vi "示波器new.vi"() -> ()   [LabVIEW 2018]
uses:
  Tektronix DPO MSO 2000 4000 Series/Tektronix DPO MSO 2000 4000 Series.lvlib
panel:
  out "Waveform Graph":waveform(dbl)(graph)
  in  "Trigger Level (0.0 V)":dbl
  in  "Timebase (0.0005 s)":dbl=0.0005 format="%#_13g"
  in  "电压 范围":dbl=10.0 format="%#_13g"
  in  "偏置 (0.0 V)":dbl
  in  "VISA Resource Name":refnum<visa-resource-name>="TCPIP::192.168.129.100::INSTR"
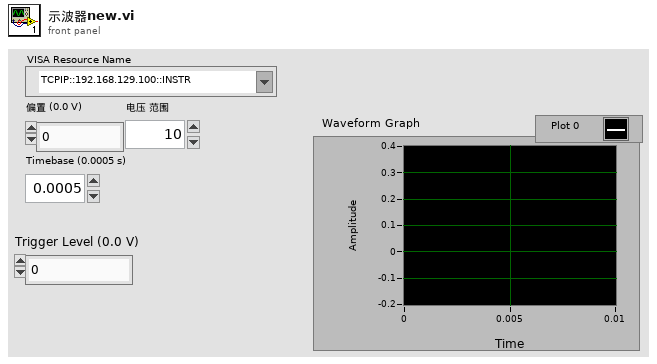
[diagram p1: front panel]
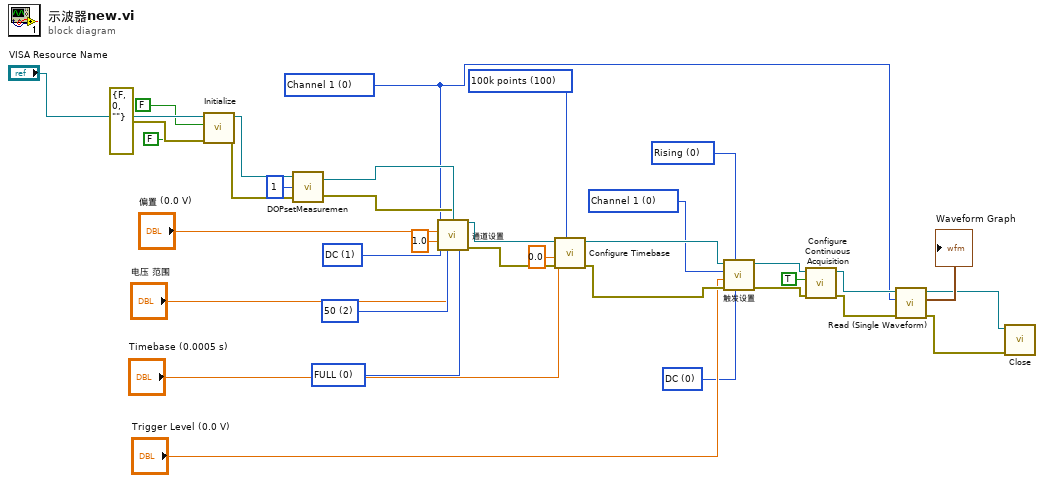
[diagram p0: block diagram]
diagram:
  w10 = u16 0 items=["DC", "HF Reject", "LF Reject", "Noise Reject", "AC"] ("Trigger Coupling (0 : DC)")
  w11 = u16 0 items=["Rising", "Falling", "Either"] ("Trigger Slope (0: Rising)")
  w13 = u16 0 items=["Channel 1", "Channel 2", "Channel 3", "Channel 4", "AC Line", "Aux", "Digital Channel 0", "Digital Channel 1", "Digital Channel 2", "Digital Channel 3", "Digital Channel 4", "Digital Channel 5", "Digital Channel 6", "Digital Channel 7", "Digital Channel 8", "Digital Channel 9", "Digital Channel 10", "Digital Channel 11", "Digital Channel 12", "Digital Channel 13", "Digital Channel 14", "Digital Channel 15", "RF"] ("Trigger Source (0: Channel 1)")
  w16 = u32 100 items=["1000 points"=1, "10k points"=10, "100k points"=100, "1M points"=1000, "5M points"=5000, "10M points"=10000] ("Record Length (10: 10k points)")
  w21 = u16 0 items=["FULL", "250 MHz", "150 MHz", "20 MHz"] ("带宽 (0: FULL)")
  w23 = u16 2 items=["1M", "75", "50"] ("输入阻抗 (0: 1M ohm)")
  w24 = u16 1 items=["AC", "DC", "Ground"] ("耦合(1: DC)")
  w4 = u16 0 items=["Channel 1", "Channel 2", "Channel 3", "Channel 4", "Math", "Reference 1", "Reference 2", "Reference 3", "Reference 4", "Bus 1", "Bus 2"] ("Channel (0: Channel 1)")
  n1 = call "Initialize.vi"("error in (no error)"=errorcluster {"status"=FALSE, "code"=0, "source"=""}, "Reset (True)"=FALSE, "ID Query (True)"=FALSE, "VISA resource name"="VISA Resource Name") -> ("error out"=w30:errorcluster, "VISA resource name out"=w31:refnum<visa-resource-name>)  [unwired: 6 in]
  n2 = call "DOPsetMeasuremen.vi"("error in (no error)"=w30, "CH"=u8 1, "VISA resource name"=w31) -> ("error out"=w27:errorcluster, "VISA resource name out"=w28:refnum<visa-resource-name>)
  n3 = call "通道设置.vi"("Channel (0: Channel 1)"=w4, "范围 (10.0 V)"="电压 范围", "VISA resource name"=w28, "带宽 (0: FULL)"=w21, "偏置 (0.0 V)"="偏置 (0.0 V)", "衰减 (1)"=1.0, "耦合(1: DC)"=w24, "输入阻抗 (0: 1M ohm)"=w23, "error in (no error)"=w27) -> ("VISA resource name out"=w20:refnum<visa-resource-name>, "error out"=w19:errorcluster)  [unwired: 5 in]
  n4 = call "Configure Timebase.vi"("Record Length (10: 10k points)"=w16, "error in (no error)"=w19, "Position (10 %)"=0.0, "Timebase (0.0005 s)"="Timebase (0.0005 s)", "VISA resource name"=w20) -> ("error out"=w14:errorcluster, "VISA resource name out"=w15:refnum<visa-resource-name>)  [unwired: 5 in]
  n5 = call "触发设置.vi"("Trigger Coupling (0 : DC)"=w10, "Trigger Slope (0: Rising)"=w11, "error in (no error)"=w14, "Trigger Level (0.0 V)"="Trigger Level (0.0 V)", "Trigger Source (0: Channel 1)"=w13, "VISA resource name"=w15) -> ("error out"=w8:errorcluster, "VISA resource name out"=w9:refnum<visa-resource-name>)  [unwired: 4 in]
  n6 = call "Configure Continuous Acquisition.vi"("error in (no error)"=w8, "Enable Continuous Acquisition Mode (T: Enable)"=TRUE, "VISA resource name"=w9) -> ("error out"=w5:errorcluster, "VISA resource name out"=w6:refnum<visa-resource-name>)  [unwired: 7 in]
  n7 = call "Read (Single Waveform).vi"("error in (no error)"=w5, "Channel (0: Channel 1)"=w4, "VISA resource name"=w6) -> ("error out"=w1:errorcluster, "Waveform Graph"=→"Waveform Graph":waveform(dbl), "VISA resource name out"=w2:refnum<visa-resource-name>)  [unwired: 6 in]
  n8 = call "Close.vi"("error in (no error)"=w1, "VISA resource name"=w2) -> ()  [unwired: 9 in, 1 out]
